vi "Zykluslängen(SubVI).vi"(1 "Formatierung":string="%d", 2 "Daten":string, 3 "Modulname":string="%d") -> (6 "Ausgang":string, 7 "Sperre":bool)   [LabVIEW 2010]
panel:
  out "aktuell 4":dbl
  in  "Zykluslänge Mod 2b (s)":dbl
  out "aktuell 3":dbl
  in  "Zykluslänge Mod 2a (s)":dbl
  out "Fehlermeldung":string="Zykluslänge muss >0 sein"
  in  "löschen":bool
  out "aktuell 2":dbl
  out "aktuell 1":dbl
  out "aktuell 0":dbl
  in  "Werte ändern":bool
  in  "Zykluslänge Mod 1a (s)":dbl
  in  "Zykluslänge Mod 1b (s)":dbl
  in  "Zykluslänge Mod 0 (s)":dbl
  in  "Zurück":bool
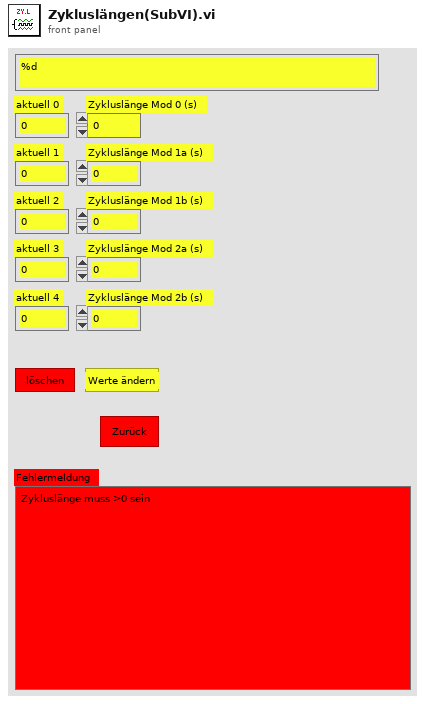
[diagram p1: front panel]
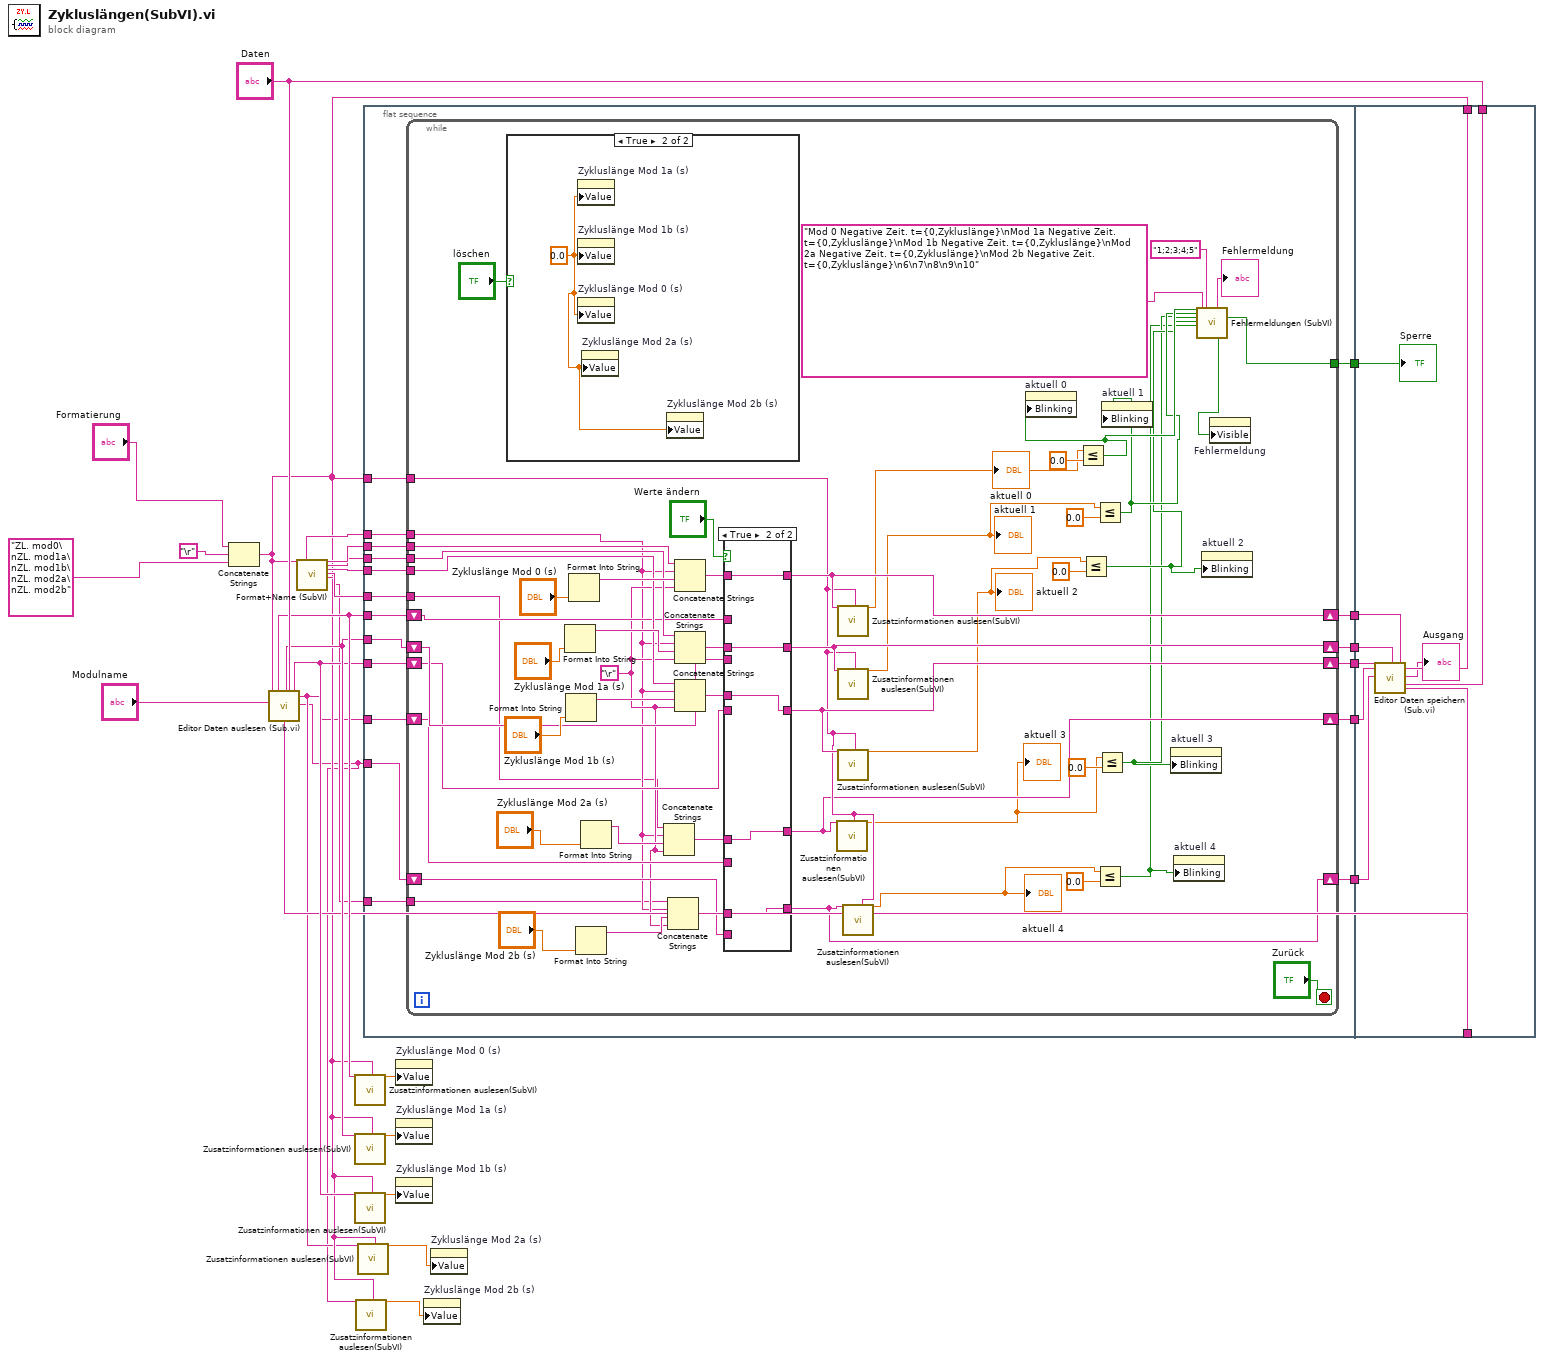
[diagram p0: block diagram]
diagram:
  n1 = Concatenate Strings("Formatierung", "\r", "ZL. mod0\nZL. mod1a\nZL. mod1b\nZL. mod2a\nZL. mod2b") -> (w5:string)
  n2 = call "Editor Daten auslesen (Sub.vi).vi"("Daten"="Daten", "Formatierung+Namen"=w5, "Modulname"="Modulname") -> ("Z 1"=w18:string, "Z 2"=w17:string, "Z 3"=w16:string, "Z 4"=w4:string, "Z5"=w3:string)  [unwired: 3 in, 17 out]
  n3 = call "Format+Name (SubVI).vi"("Format+Namen Eingang"=w5) -> ("Trennzeichen"=w27:string, "1"=w28:string, "2"=w26:string, "3"=w25:string, "4"=w7:string, "5"=w6:string)  [unwired: 15 in, 6 out]
  n4 = call "Zusatzinformationen auslesen(SubVI).vi"("Zusatzinformationen"=w18, "Format+Namen"=w5) -> ("1"=w15:dbl)  [unwired: 18 in, 7 out]
  n5 = call "Zusatzinformationen auslesen(SubVI).vi"("Zusatzinformationen"=w17, "Format+Namen"=w5) -> ("1"=w14:dbl)  [unwired: 18 in, 7 out]
  n6 = call "Zusatzinformationen auslesen(SubVI).vi"("Zusatzinformationen"=w16, "Format+Namen"=w5) -> ("1"=w13:dbl)  [unwired: 18 in, 7 out]
  n7 = call "Zusatzinformationen auslesen(SubVI).vi"("Zusatzinformationen"=w3, "Format+Namen"=w5) -> ("1"=w1:dbl)  [unwired: 18 in, 7 out]
  n8 = call "Zusatzinformationen auslesen(SubVI).vi"("Zusatzinformationen"=w4, "Format+Namen"=w5) -> ("1"=w2:dbl)  [unwired: 18 in, 7 out]
  n9 = flat-sequence {
    tunnel: w28 -> [w46]
    tunnel: w27 -> [w45]
    tunnel: w26 -> [w44]
    tunnel: w25 -> [w43]
    tunnel: [w42] -> w22
    tunnel: w18 -> [w41]
    tunnel: [w40] -> w21
    tunnel: w17 -> [w39]
    tunnel: [w38] -> w20
    tunnel: w16 -> [w37]
    tunnel: w5 -> [w36]
    tunnel: [w35] -> w10
    tunnel: w4 -> [w34]
    tunnel: w3 -> [w33]
    tunnel: [w32] -> w9
    tunnel: [w31] -> w8
    tunnel: w7 -> [w30]
    tunnel: w6 -> [w29]
    tunnel: w5 -> [w123]
    tunnel: w22 -> [w121]
    tunnel: w21 -> [w120]
    tunnel: w20 -> [w119]
    tunnel: "Daten" -> [w118]
    tunnel: "Modulname" -> [w117]
    tunnel: w10 -> [w116]
    tunnel: w9 -> [w115]
    tunnel: w8 -> [w114]
    frame #0 {
      n10 = while {
        tunnel: w46 -> [w101]
        tunnel: w45 -> [w55]
        tunnel: w44 -> [w94]
        tunnel: w43 -> [w93]
        shift-right: [w85] -> w42
        shift-left: w41 -> [w91]
        shift-right: [w84] -> w40
        shift-left: w39 -> [w90]
        shift-right: [w83] -> w38
        shift-left: w37 -> [w89]
        tunnel: w36 -> [w67]
        tunnel: [w71] -> w35
        shift-right: [w62] -> w32
        shift-left: w34 -> [w64]
        shift-right: [w61] -> w31
        shift-left: w33 -> [w63]
        tunnel: w30 -> [w54]
        tunnel: w29 -> [w53]
        stop <- "Zurück" stop-if-true
        w56 = "\r"
        n11 = case shown="True" "löschen" {
          frame False {
          }
          frame True {
            w103 = 0.0 ("Zykluslänge Mod 1 (s)")
            n12 = property on="Zykluslänge Mod 1a (s)" class="DigWert (strikt)"("Value"=w103) -> ()  [unwired: 2 in, 2 out]
            n13 = property on="Zykluslänge Mod 1b (s)" class="DigWert (strikt)"("Value"=w103) -> ()  [unwired: 2 in, 2 out]
            n14 = property on="Zykluslänge Mod 0 (s)" class="DigWert (strikt)"("Value"=w103) -> ()  [unwired: 2 in, 2 out]
            n15 = property on="Zykluslänge Mod 2a (s)" class="DigWert (strikt)"("Value"=w103) -> ()  [unwired: 2 in, 2 out]
            n16 = property on="Zykluslänge Mod 2b (s)" class="DigWert (strikt)"("Value"=w103) -> ()  [unwired: 2 in, 2 out]
          }
        }
        n17 = Format Into String("Zykluslänge Mod 1a (s)") -> (resulting string=w97:string)  [unwired: 3 in, 1 out]
        n18 = Format Into String("Zykluslänge Mod 1b (s)") -> (resulting string=w96:string)  [unwired: 3 in, 1 out]
        n19 = Format Into String("Zykluslänge Mod 0 (s)") -> (resulting string=w99:string)  [unwired: 3 in, 1 out]
        n20 = Format Into String("Zykluslänge Mod 2b (s)") -> (resulting string=w58:string)  [unwired: 3 in, 1 out]
        n21 = Format Into String("Zykluslänge Mod 2a (s)") -> (resulting string=w57:string)  [unwired: 3 in, 1 out]
        n22 = Concatenate Strings(w54, w55, w57, w56) -> (w66:string)
        n23 = Concatenate Strings(w53, w55, w58, w56) -> (w65:string)
        n24 = Concatenate Strings(w101, w55, w99, w56) -> (w88:string)
        n25 = Concatenate Strings(w94, w55, w97, w56) -> (w87:string)
        n26 = Concatenate Strings(w93, w55, w96, w56) -> (w86:string)
        n27 = case shown="True" "Werte ändern" {
          tunnel: [w108 w113] -> w85
          tunnel: w91 -> [w108 _]
          tunnel: [w107 w112] -> w84
          tunnel: w90 -> [w107 _]
          tunnel: [w106 w111] -> w83
          tunnel: w89 -> [w106 _]
          tunnel: w88 -> [_ w113]
          tunnel: w87 -> [_ w112]
          tunnel: w86 -> [_ w111]
          tunnel: [w105 w110] -> w62
          tunnel: w66 -> [_ w110]
          tunnel: [w104 w109] -> w61
          tunnel: w65 -> [_ w109]
          tunnel: w64 -> [w105 _]
          tunnel: w63 -> [w104 _]
          frame False {
          }
          frame True {
          }
        }
        n28 = call "Zusatzinformationen auslesen(SubVI).vi"("Zusatzinformationen"=w62, "Format+Namen"=w67) -> ("1"=w50:dbl)  [unwired: 18 in, 7 out]
        "aktuell 3" <- w50
        n29 = call "Zusatzinformationen auslesen(SubVI).vi"("Zusatzinformationen"=w85, "Format+Namen"=w67) -> ("1"=w80:dbl)  [unwired: 18 in, 7 out]
        "aktuell 0" <- w80
        n30 = call "Zusatzinformationen auslesen(SubVI).vi"("Zusatzinformationen"=w84, "Format+Namen"=w67) -> ("1"=w77:dbl)  [unwired: 18 in, 7 out]
        "aktuell 1" <- w77
        n31 = call "Zusatzinformationen auslesen(SubVI).vi"("Zusatzinformationen"=w83, "Format+Namen"=w67) -> ("1"=w76:dbl)  [unwired: 18 in, 7 out]
        "aktuell 2" <- w76
        n32 = call "Zusatzinformationen auslesen(SubVI).vi"("Zusatzinformationen"=w61, "Format+Namen"=w67) -> ("1"=w49:dbl)  [unwired: 18 in, 7 out]
        "aktuell 4" <- w49
        n33 = Less Or Equal?(x=w80, y=0.0) -> (x <= y?=w70:bool)
        n34 = property on="aktuell 0" class="DigWert (strikt)"("Blinking"=w70) -> ()  [unwired: 2 in, 2 out]
        n35 = Less Or Equal?(x=w76, y=0.0) -> (x <= y?=w68:bool)
        n36 = Less Or Equal?(x=w77, y=0.0) -> (x <= y?=w69:bool)
        n37 = Less Or Equal?(x=w49, y=0.0) -> (x <= y?=w47:bool)
        n38 = Less Or Equal?(x=w50, y=0.0) -> (x <= y?=w48:bool)
        n39 = property on="aktuell 1" class="DigWert (strikt)"("Blinking"=w69) -> ()  [unwired: 2 in, 2 out]
        n40 = property on="aktuell 3" class="DigWert (strikt)"("Blinking"=w48) -> ()  [unwired: 2 in, 2 out]
        n41 = property on="aktuell 4" class="DigWert (strikt)"("Blinking"=w47) -> ()  [unwired: 2 in, 2 out]
        n42 = call "Fehlermeldungen (SubVI).vi"("Fehler 1"=w70, "Fehler 2"=w69, "Fehler 3"=w68, "Fehler 4"=w48, "Fehler 5"=w47, "Fehlermeldungen Namen"="Mod 0 Negative Zeit. t={0,Zykluslänge}\nMod 1a Negative Zeit. t={0,Zykluslänge}\nMod 1b Negative Zeit. t={0,Zykluslänge}\nMod 2a Negative Zeit. t={0,Zykluslänge}\nMod 2b Negative Zeit. t={0,Zykluslänge}\n6\n7\n8\n9\n10", "Kritischefehler Positionen"="1;2;3;4;5") -> ("Fehlermeldung Ausgang"=→"Fehlermeldung":string, "Fehler?"=w72:bool, "Sperre"=w71:bool)  [unwired: 18 in]
        n43 = property on="aktuell 2" class="DigWert (strikt)"("Blinking"=w68) -> ()  [unwired: 2 in, 2 out]
        n44 = property on="Fehlermeldung" class="Str"("Visible"=w72) -> ()  [unwired: 2 in, 2 out]
      }
    }
    frame #1 {
      n45 = call "Editor Daten speichern (Sub.vi).vi"("Z 4"=w115, "Z 5"=w114, "Z 3"=w119, "Z 2"=w120, "Z 1"=w121, "Formatierung+Namen"=w123, "Daten"=w118, "Modulname"=w117) -> ("Ausgang"=→"Ausgang":string)  [unwired: 19 in]
      "Sperre" <- w116
    }
  }
  n46 = property on="Zykluslänge Mod 0 (s)" class="DigWert (strikt)"("Value"=w15) -> ()  [unwired: 2 in, 2 out]
  n47 = property on="Zykluslänge Mod 1a (s)" class="DigWert (strikt)"("Value"=w14) -> ()  [unwired: 2 in, 2 out]
  n48 = property on="Zykluslänge Mod 1b (s)" class="DigWert (strikt)"("Value"=w13) -> ()  [unwired: 2 in, 2 out]
  n49 = property on="Zykluslänge Mod 2b (s)" class="DigWert (strikt)"("Value"=w1) -> ()  [unwired: 2 in, 2 out]
  n50 = property on="Zykluslänge Mod 2a (s)" class="DigWert (strikt)"("Value"=w2) -> ()  [unwired: 2 in, 2 out]
